vi "APX VarianTMP HPC.vi"() -> ()   [LabVIEW 2015]
uses:
  <vilib>/Instr/_visa.llb/VISA Configure Serial Port (Instr).vi
  <userlib>/caLab/Private/Get_PV-1D.vi
  <userlib>/caLab/Private/Put_DBL_PV.vi
  <userlib>/caLab/Private/Put_DBL-1D_PV-1D.vi
panel:
  in  "stop":bool
  out "APX:HPCTurboS":dbl
  out "APX:HPCTrubo_STOP":bool
  out "APX:HPCTurbo_START":bool
  out "SERIAL":string
  out "V-81":refnum<visa-resource-name>="COM4"
  out "APX:HPCTurboF":dbl caption="F_20/Hz"
  out "APX:HPCTurboP":dbl caption="P_20/W"
  out "APX:HPCTurboS:STR":string
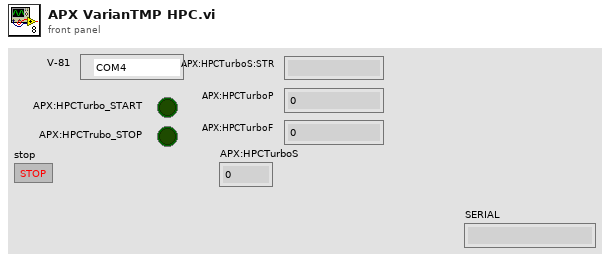
[diagram p1: front panel]
types:
  T1 = enum16{"START", "STOP", "REMOTE/SERIAL", "REMOTE", "SERIAL", "START/STOP", "PUMP STATUS", "Driving Frequency", "PUMP POWER", "PRESSURE"}
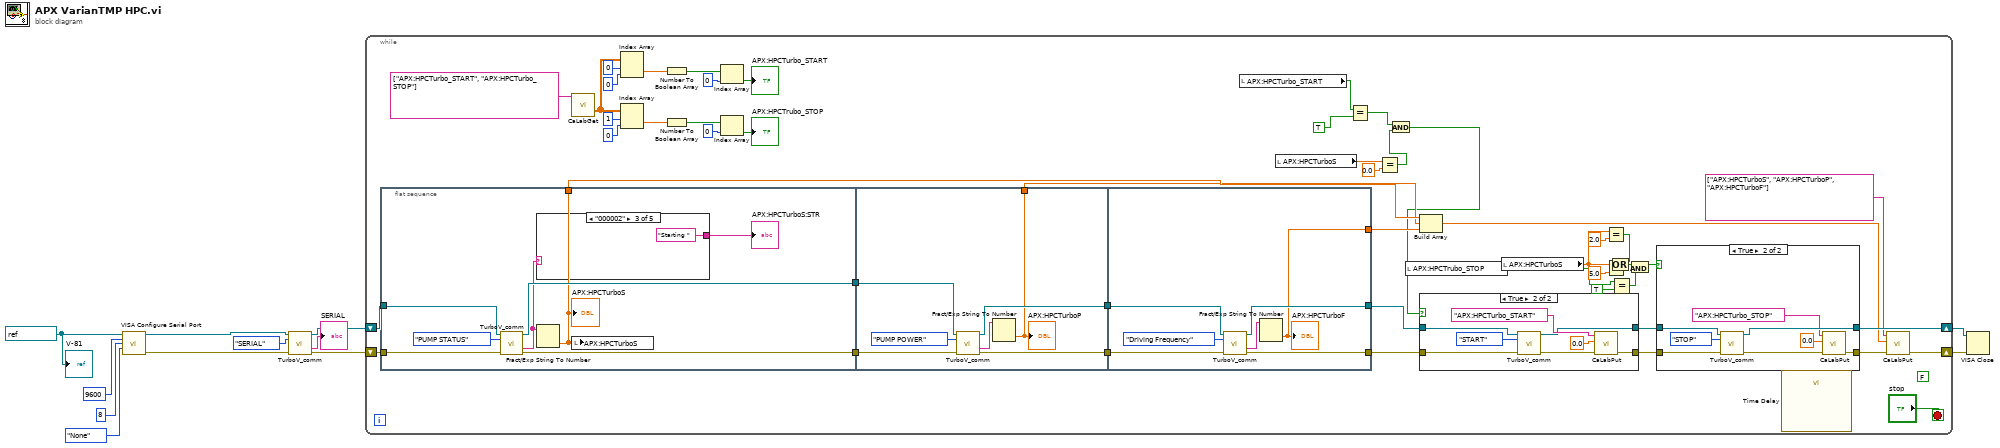
[diagram p0: block diagram]
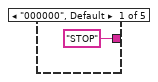
[diagram p2: hidden frame]
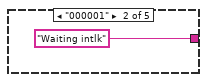
[diagram p3: hidden frame]
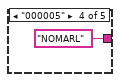
[diagram p4: hidden frame]
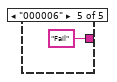
[diagram p5: hidden frame]
diagram:
  w12 = refnum<visa-resource-name> "COM25" ("VISA resource name")
  n1 = call-poly "VISA Configure Serial Port"("VISA resource name"=w12, "baud rate (9600)"=u32 9600, "data bits (8)"=u16 8, "parity (0:none)"=enum16{"None", "Odd", "Even", "Mark", "Space"}."None") -> ("VISA resource name out"=w5:refnum<visa-resource-name>, "error out"=w3:errorcluster)  [unwired: 10 in]
  n2 = call "TurboV_comm.vi"("VISA resource name"=w5, "Command"=T1."SERIAL", "error in (no error)"=w3) -> ("VISA resource name out"=w4:refnum<visa-resource-name>, "read buffer"=→"SERIAL":string, "error out"=w2:errorcluster)  [unwired: 10 in]
  n3 = while {
    shift-right: [w58] -> w8
    shift-left: w4 -> [w56]
    shift-right: [w57] -> w7
    shift-left: w2 -> [w55]
    stop <- "stop" stop-if-true
    (unwired) FALSE
    n4 = flat-sequence {
      tunnel: w56 -> [w70]
      tunnel: w55 -> [w69]
      tunnel: [w68] -> w62
      tunnel: [w67] -> w61
      tunnel: [w63] -> w53
      tunnel: w62 -> [w81]
      tunnel: w61 -> [w78]
      tunnel: [w80] -> w60
      tunnel: [w79] -> w59
      tunnel: [w76] -> w52
      tunnel: w60 -> [w89]
      tunnel: w59 -> [w88]
      tunnel: [w85] -> w26
      tunnel: [w84] -> w27
      tunnel: [w83] -> w51
      frame #0 {
        n5 = call "TurboV_comm.vi"("VISA resource name"=w70, "Command"=T1."PUMP STATUS", "error in (no error)"=w69) -> ("VISA resource name out"=w68:refnum<visa-resource-name>, "read buffer"=w64:string, "error out"=w67:errorcluster)  [unwired: 10 in]
        n6 = case shown="\"000002\"" w64 {
          tunnel: ["STOP" "Waiting intlk" "Starting " "NOMARL" "Fail"] -> w65
          frame "000000", Default {
          }
          frame "000001" {
          }
          frame "000002" {
          }
          frame "000005" {
          }
          frame "000006" {
          }
        }
        "APX:HPCTurboS:STR" <- w65
        n7 = Fract/Exp String To Number(string=w64) -> (number=w63:dbl)  [unwired: 3 in, 1 out]
        "APX:HPCTurboS" <- w63
        n8 = local write "APX:HPCTurboS"(w63) -> ()
      }
      frame #1 {
        n9 = call "TurboV_comm.vi"("VISA resource name"=w81, "Command"=T1."PUMP POWER", "error in (no error)"=w78) -> ("VISA resource name out"=w80:refnum<visa-resource-name>, "read buffer"=w77:string, "error out"=w79:errorcluster)  [unwired: 10 in]
        n10 = Fract/Exp String To Number(string=w77) -> (number=w76:dbl)  [unwired: 3 in, 1 out]
        "APX:HPCTurboP" <- w76
      }
      frame #2 {
        n11 = call "TurboV_comm.vi"("VISA resource name"=w89, "Command"=T1."Driving Frequency", "error in (no error)"=w88) -> ("VISA resource name out"=w84:refnum<visa-resource-name>, "read buffer"=w86:string, "error out"=w85:errorcluster)  [unwired: 10 in]
        n12 = Fract/Exp String To Number(string=w86) -> (number=w83:dbl)  [unwired: 3 in, 1 out]
        "APX:HPCTurboF" <- w83
      }
    }
    n13 = call-poly "CaLabGet.vi"("PV Names"=string[] ["APX:HPCTurbo_START", "APX:HPCTurbo_STOP"]) -> ("Value Array (number)"=w37:dbl[][])  [unwired: 8 in, 6 out]
    n14 = Index Array(array=w37, index (row)=0 ("disabled index (row)"), index (col)=0 ("index (row)")) -> (element=w44:dbl)
    n15 = Index Array(array=w37, index (row)=1 ("disabled index (row)"), index (col)=0 ("index (row)")) -> (element=w38:dbl)
    n16 = Number To Boolean Array(number=w44) -> (Boolean array=w46:bool[])
    n17 = Number To Boolean Array(number=w38) -> (Boolean array=w40:bool[])
    n18 = Index Array(array=w46, index=0) -> (element=→"APX:HPCTurbo_START":bool)
    n19 = Index Array(array=w40, index=0) -> (element=→"APX:HPCTrubo_STOP":bool)
    n20 = local read "APX:HPCTurbo_START"() -> (w13:bool)
    n21 = local read "APX:HPCTurboS"() -> (w34:dbl)
    n22 = Equal?(x=w13, y=TRUE) -> (x = y?=w15:bool)
    n23 = Equal?(x=w34, y=0.0) -> (x = y?=w17:bool)
    n24 = And(x=w15, y=w17) -> (x .and. y?=w16:bool)
    n25 = local read "APX:HPCTrubo_STOP"() -> (w19:bool)
    n26 = Build Array(w53, w52, w51) -> (w50:dbl[])
    n27 = case shown="True" w16 {
      tunnel: [w101 w103] -> w24
      tunnel: w27 -> [w100 w108]
      tunnel: w26 -> [w101 w107]
      tunnel: [w100 w102] -> w25
      frame False {
      }
      frame True {
        n28 = call "TurboV_comm.vi"("VISA resource name"=w108, "Command"=T1."START", "error in (no error)"=w107) -> ("VISA resource name out"=w102:refnum<visa-resource-name>, "error out"=w104:errorcluster)  [unwired: 10 in, 1 out]
        n29 = call-poly <userlib>:"CaLabPut.vi"("Error in (no error)"=w104, "Value"=0.0, "PV Name"="APX:HPCTurbo_START") -> ("Error out"=w103:errorcluster)  [unwired: 5 in, 3 out]
      }
    }
    n30 = local read "APX:HPCTurboS"() -> (w30:dbl)
    n31 = Equal?(x=w30, y=2.0) -> (x = y?=w31:bool)
    n32 = Equal?(x=w30, y=5.0) -> (x = y?=w32:bool)
    n33 = Or(x=w31, y=w32) -> (x .or. y?=w33:bool)
    n34 = Equal?(x=w19, y=TRUE) -> (x = y?=w20:bool)
    n35 = And(x=w33, y=w20) -> (x .and. y?=w21:bool)
    n36 = case shown="True" w21 {
      tunnel: [w91 w99] -> w58
      tunnel: [w90 w92] -> w23
      tunnel: w25 -> [w91 w98]
      tunnel: w24 -> [w90 w97]
      frame False {
      }
      frame True {
        n37 = call "TurboV_comm.vi"("VISA resource name"=w98, "Command"=T1."STOP", "error in (no error)"=w97) -> ("VISA resource name out"=w99:refnum<visa-resource-name>, "error out"=w93:errorcluster)  [unwired: 10 in, 1 out]
        n38 = call-poly <userlib>:"CaLabPut.vi"("Error in (no error)"=w93, "Value"=0.0, "PV Name"="APX:HPCTurbo_STOP") -> ("Error out"=w92:errorcluster)  [unwired: 5 in, 3 out]
      }
    }
    n39 = call "Time Delay"() -> ()  [unwired: 11 in, 1 out]
    n40 = call-poly <userlib>:"CaLabPut.vi"("Error in (no error)"=w23, "Values"=w50, "PV Names"=string[] ["APX:HPCTurboS", "APX:HPCTurboP", "APX:HPCTurboF"]) -> ("Error out"=w57:errorcluster)  [unwired: 5 in, 3 out]
  }
  n41 = VISA Close(VISA resource name=w8, error in (no error)=w7) -> ()  [unwired: 1 out]
  "V-81" <- w12
